vi "Message Event Global.vi"(8 "error in (no error)":errorcluster, 9 "Clear (F)":bool, 10 "Set (F)":bool, 11 "Message Event in":refnum<user-event>) -> (0 "error out":errorcluster, 1 "Is Set?":bool, 2 "Succeeded?":bool, 3 "Message Event out":refnum<user-event>)   [LabVIEW 2020, in "Caraya.lvlib" / "Basic Test Manager.lvclass"]
uses:
  Basic Test Manager.lvclass
  Test Manager Message/TestManagerMsg.lvclass
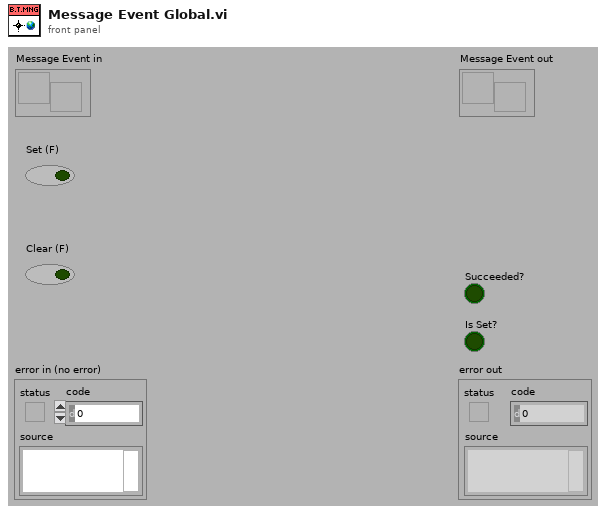
[diagram p1: front panel]
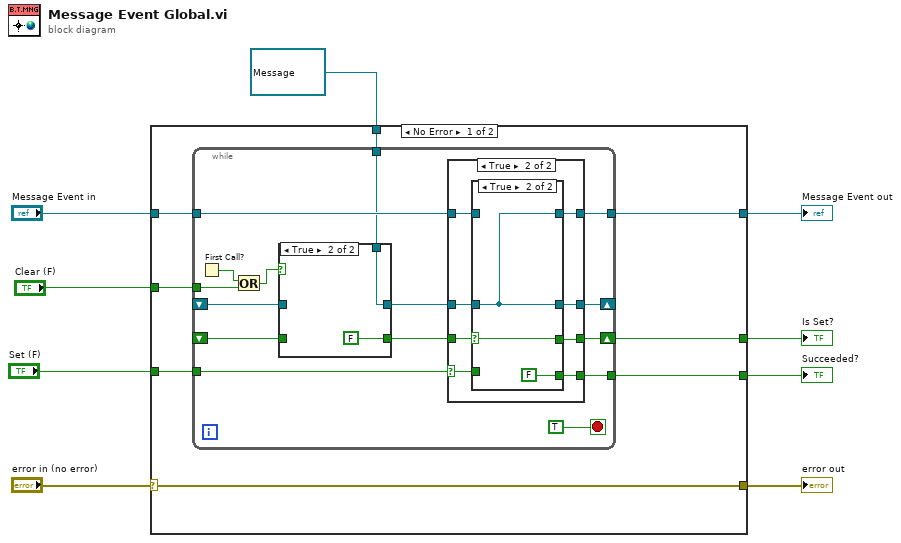
[diagram p0: block diagram]
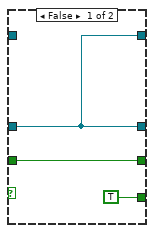
[diagram p3: hidden frame]
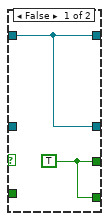
[diagram p4: hidden frame]
diagram:
  n1 = case shown="No Error" "error in (no error)" {
    selector: "error in (no error)" -> [w15 w53]
    tunnel: "Message Event in" -> [w17 w54]
    tunnel: "Set (F)" -> [w16 _]
    tunnel: [w14 w54] -> w6
    tunnel: [w15 w53] -> w5
    tunnel: [w13 _] -> w4
    tunnel: [w12 _] -> w3
    tunnel: refnum<user-event> refnum ("Message Event in") -> [w11 _]
    tunnel: "Clear (F)" -> [w10 _]
    frame No Error {
      n2 = while {
        tunnel: w16 -> [w31]
        tunnel: w17 -> [w29]
        shift-right: [w27] -> _
        shift-left: _ -> [w30]
        tunnel: [w26] -> w14
        shift-right: [w24] -> w13
        shift-left: _ -> [w25]
        tunnel: [w22] -> w12
        tunnel: w11 -> [w21]
        tunnel: w10 -> [w20]
        stop <- TRUE stop-if-true
        n3 = First Call?() -> (First Call?: T/F=w19:bool)
        n4 = Or(x=w19, y=w20) -> (x .or. y?=w18:bool)
        n5 = case shown="True" w18 {
          tunnel: w30 -> [w34 _]
          tunnel: [w34 w35] -> w28
          tunnel: w25 -> [w33 _]
          tunnel: [w33 FALSE] -> w23
          tunnel: w21 -> [_ w35]
          frame False {
          }
          frame True {
          }
        }
        n6 = case shown="True" w31 {
          selector: w31 -> [_ w41]
          tunnel: w29 -> [_ w47]
          tunnel: w28 -> [w39 w44]
          tunnel: [w39 w43] -> w27
          tunnel: [w39 w45] -> w26
          tunnel: [w38 w42] -> w24
          tunnel: w23 -> [w38 w46]
          tunnel: [TRUE w40] -> w22
          frame False {
          }
          frame True {
            n7 = case shown="True" w46 {
              selector: w46 -> [_ w51]
              tunnel: w47 -> [w49 _]
              tunnel: [w49 w52] -> w45
              tunnel: w44 -> [_ w52]
              tunnel: [w49 w52] -> w43
              tunnel: [w48 w51] -> w42
              tunnel: w41 -> [_ _]
              tunnel: [w48 FALSE] -> w40
              frame False {
                w48 = TRUE
              }
              frame True {
              }
            }
          }
        }
      }
    }
    frame Error {
    }
  }
  "error out" <- w5
  "Message Event out" <- w6
  "Is Set?" <- w4
  "Succeeded?" <- w3
